vi "Get Property Values (Numeric Property).vi"(1 "data type":dbl[](array[numeric]), 5 "property":T2 {"data type" items=["Unknown"=0, "String"=23, "I32"=3, "I64"=4, "DBL"=10, "Time stamp"=30]; "object type" items=["File", "Channel Group", "Channel"]}, 7 "result references":T1[](array[typedef]), 11 "error in (no error)":errorcluster) -> (6 "property values":dbl[](array[numeric]), 8 "result references out":T1[](array[typedef]), 15 "error out":errorcluster)   [LabVIEW 2020, in "NI_DataFinder.lvlib"]
doc: "Determines from the result references the values of a numeric property."
uses:
  <vilib>/DataFinder/NI_DataFinder.lvlib
  <vilib>/DataFinder/DataTypes/property.ctl
  <vilib>/DataFinder/DataTypes/object type.ctl
  <vilib>/DataFinder/DataTypes/data type.ctl
  <vilib>/userdefined/DFSearchResult.ctl
  <vilib>/userdefined/NI_DataFinder Controls.lvlib
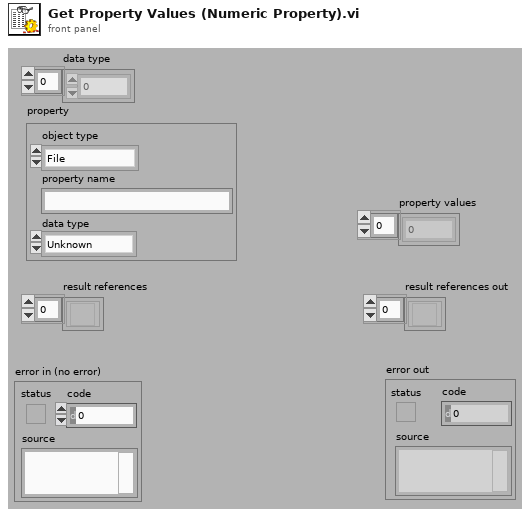
[diagram p1: front panel]
types:
  T1 = typedef "NI_DataFinder Controls.lvlib/DFSearchResult.ctl" = refnum<k20>
  T2 = typedef "NI_DataFinder.lvlib/property.ctl" = cluster{"object type":T3, "property name":string, "data type":T4}
  T3 = typedef "NI_DataFinder.lvlib/object type.ctl" = u16
  T4 = typedef "NI_DataFinder.lvlib/data type.ctl" = u16
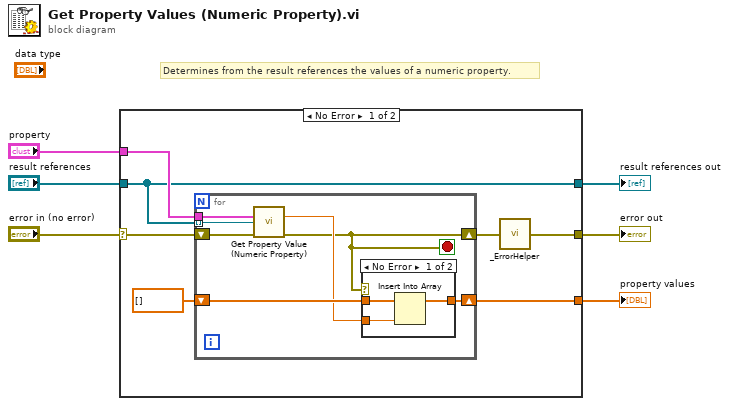
[diagram p0: block diagram]
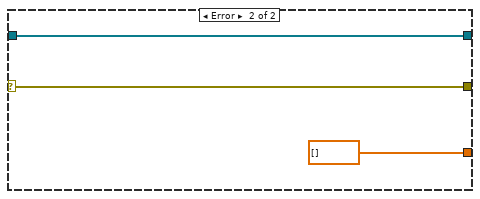
[diagram p3: hidden frame]
diagram:
  # "Determines from the result references the values of a numeric property."
  n1 = case shown="No Error" "error in (no error)" {
    selector: "error in (no error)" -> [w13 w27]
    tunnel: [w10 w27] -> w4
    tunnel: "result references" -> [w7 w26]
    tunnel: [w12 dbl[] []] -> w3
    tunnel: "property" -> [w11 _]
    tunnel: [w7 w26] -> w1
    frame No Error {
      n2 = for {
        tunnel: w7 -> [w18] mode=indexing
        tunnel: w11 -> [w17]
        shift-right: [w14] -> w9
        shift-left: w13 -> [w16]
        shift-right: [w19] -> w12
        shift-left: dbl[] [] -> [w20]
        stop <- w14 stop-if-true
        n3 = call <vilib>:"Get Property Value (Numeric Property).vi"("property"=w17, "result reference"=w18, "error in (no error)"=w16) -> ("property value"=w15:dbl, "error out"=w14:errorcluster)  [unwired: 10 in, 1 out]
        n4 = case shown="No Error" w14 {
          tunnel: w20 -> [w23 w24]
          tunnel: w15 -> [w22 _]
          tunnel: [w21 w24] -> w19
          frame No Error {
            n5 = Insert Into Array(array=w23, new element=w22) -> (w21:dbl[])  [unwired: 1 in]
          }
          frame Error {
          }
        }
      }
      n6 = call <vilib>:"_ErrorHelper.vi"("error IO"=w9) -> ("error out"=w10:errorcluster)
    }
    frame Error {
    }
  }
  "error out" <- w4
  "property values" <- w3
  "result references out" <- w1
